vi "Force Remove Item.vi"(8 "error in":errorcluster, 11 "item ref":u64) -> (0 "error out":errorcluster)   [LabVIEW 2027, in "Custom Device Serialization.lvlib"]
uses:
  Custom Device Serialization.lvlib
  System Explorer Action.ctl
  C:/NetCoreDLL/NationalInstruments.VeriStand.SystemStorage.dll
  NetCoreDLL/NationalInstruments.VeriStand.SystemStorage.dll
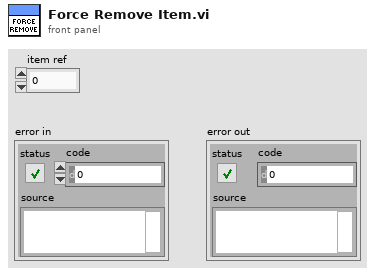
[diagram p1: front panel]
types:
  T1 = typedef "Custom Device Serialization.lvlib/System Explorer Action.ctl" = u16
  T2 = typedef "Custom Device API.lvlib/Custom Device Item Ref.ctl" = u64
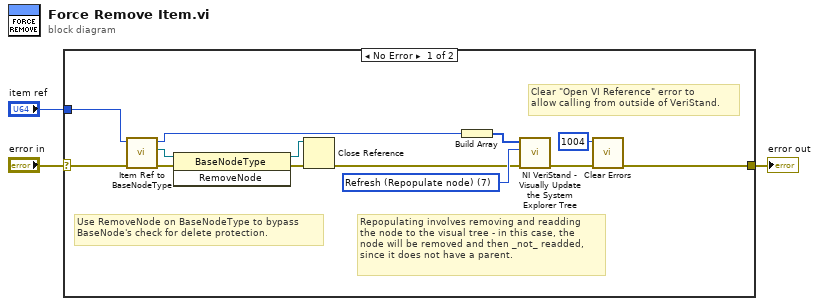
[diagram p0: block diagram]
diagram:
  n1 = case shown="No Error" "error in" {
    selector: "error in" -> [w8 w17]
    tunnel: [w9 w17] -> w3
    tunnel: "item ref" -> [w7 _]
    frame No Error {
      w13 = T1 7 items=["Refresh (Add)"=5, "Refresh (Repopulate node)"=7, "Refresh (Delete)"=9] ("Action")
      # "Clear \"Open VI Reference\" error to\nallow calling from outside of VeriStand."
      # "Use RemoveNode on BaseNodeType to bypass\nBaseNode's check for delete protection."
      # "Repopulating involves removing and readding\nthe node to the visual tree - in this case, the\nnode will be removed and then _not_ readded,\nsince it does not have a parent."
      n2 = call "Item Ref to BaseNodeType.vi"("error in (no error)"=w8, "item ref in"=w7) -> ("error out"=w4:errorcluster, "NationalInstruments.VeriStand.SystemStorage.BaseNodeType"=w5:refnum<k39>, "item ref out"=w6:T2)  [unwired: 7 in]
      n3 = invoke class="BaseNodeType" method="RemoveNode"(reference=w5, error in=w4) -> (reference out=w15:refnum<k39>, error out=w16:errorcluster)  [unwired: 1 in, 1 out]
      n4 = Close Reference(reference=w15, error in (no error)=w16) -> (error out=w11:errorcluster)
      n5 = Build Array(w6) -> (w14:T2[])
      n6 = call "NI VeriStand - Visually Update the System Explorer Tree.vi"("error in (no error)"=w11, "Action"=w13, "Node IDs"=w14) -> ("error out"=w10:errorcluster)  [unwired: 8 in]
      n7 = call <vilib>:"Clear Errors.vi"("error in (no error)"=w10, "specific error code to clear (0: all)"=1004) -> ("error out"=w9:errorcluster)  [unwired: 4 in, 1 out]
    }
    frame Error {
    }
  }
  "error out" <- w3
